vi "Handle Error.vi"(8 "error in (no error)":errorcluster, 11 "Factory in":refnum<class "Factory.lvclass">) -> (0 "error out":errorcluster, 3 "Factory out":refnum<class "Factory.lvclass">)   [LabVIEW 2019, in "Factory.lvclass"]
uses:
  Factory.lvclass
panel:
  in  "Close":bool
  out "Message":string
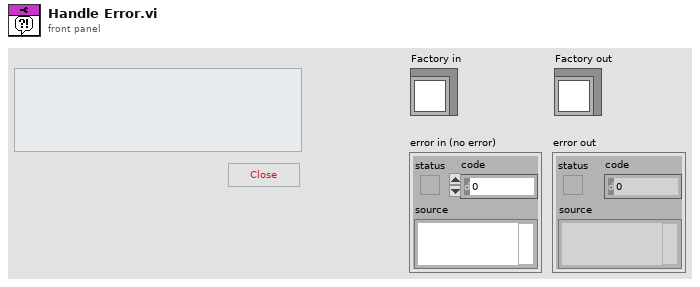
[diagram p1: front panel]
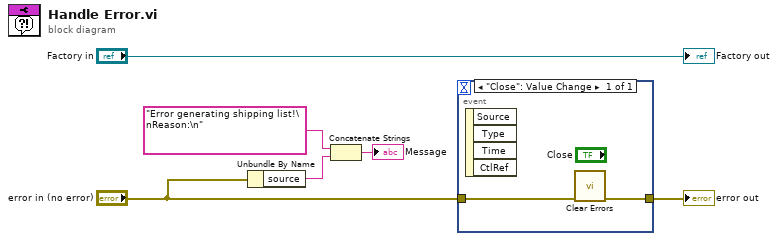
[diagram p0: block diagram]
diagram:
  n1 = Unbundle By Name("error in (no error)") -> ("source"=w4:string)
  n2 = Concatenate Strings("Error generating shipping list!\nReason:\n" ("string"), w4) -> (→"Message":string)
  n3 = event shown="[0] \"Close\": Value Change" {
    selector: _ -> [_]
    dyn-events: _ -> [_]
    timeout: _ -> [_]
    tunnel: "error in (no error)" -> [w8]
    tunnel: [w7] -> w1
    event "Close": Value Change {
      n4 = event-data() -> ()  [unwired: 1 in, 4 out]
      n5 = call <vilib>:"Clear Errors.vi"("error in (no error)"=w8) -> ("error out"=w7:errorcluster)  [unwired: 5 in, 1 out]
    }
  }
  "error out" <- w1
  "Factory out" <- "Factory in"
